vi "Configure RFSG.vi"(0 "Path in":refnum<class "SA 8GHz Path.lvclass">, 5 "Cal Point in":T1, 7 "External Gain":dbl, 9 "Digital Gain":dbl, 11 "error in (no error)":errorcluster) -> (4 "Path out":refnum<class "SA 8GHz Path.lvclass">, 6 "Cal Point out":T1, 15 "error out":errorcluster)   [LabVIEW 2023, in "RFFixtureCharact.RMM.lvlib" / "SA 8GHz Path.lvclass"]
uses:
  SA 8GHz Path.lvclass
  Public/Base Classes/Scalar/Scalar Path/Type Definitions/Cal Point.ctl
  <instrlib>/niRFSG/niRFSG.llb/niRFSG Ref Clock Sources.ctl
  SA 8GHz Path.lvclass/SA 8GHz Path.ctl
  Public/Base Classes/Scalar/Scalar Path/Scalar Path.lvclass
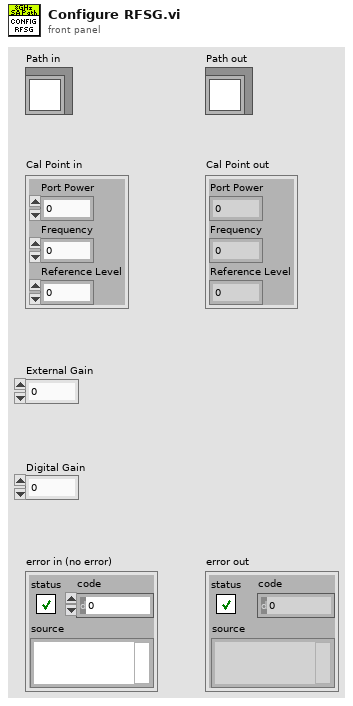
[diagram p1: front panel]
types:
  T1 = typedef "RFFixtureCharact.Public.lvlib/Scalar Path.lvclass/Cal Point.ctl" = cluster{"Port Power":dbl, "Frequency":dbl, "Reference Level":dbl}
  T2 = typedef "niRFSG Ref Clock Sources.ctl" = string
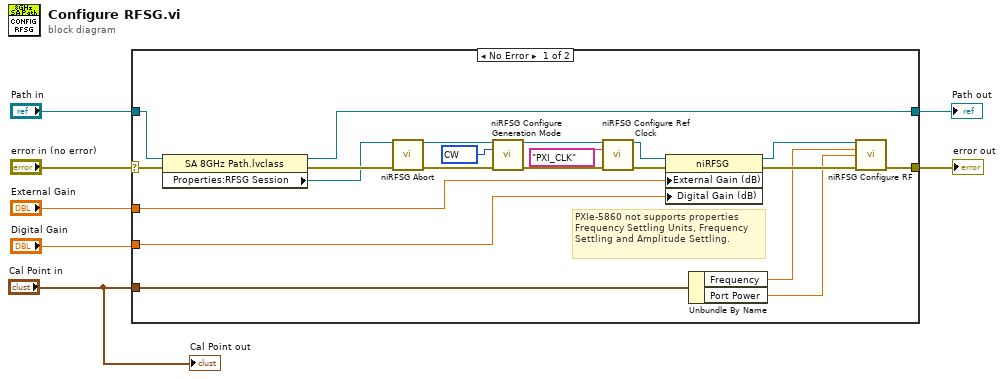
[diagram p0: block diagram]
diagram:
  n1 = case shown="No Error" "error in (no error)" {
    selector: "error in (no error)" -> [w17 w30]
    tunnel: [w18 w30] -> w4
    tunnel: [w10 w29] -> w6
    tunnel: "Path in" -> [w11 w29]
    tunnel: "Cal Point in" -> [w15 _]
    tunnel: "External Gain" -> [w12 _]
    tunnel: "Digital Gain" -> [w8 _]
    frame No Error {
      w22 = 1000 items=["CW"=1000, "Arb Waveform"=1001, "Script"=1002] ("generation mode")
      # "PXIe-5860 not supports properties Frequency Settling Units, Frequency Settling and Amplitude Settling."
      n2 = property class="SA 8GHz Path.lvclass"(reference=w11, error in=w17) -> (reference out=w10:refnum<class "SA 8GHz Path.lvclass">, error out=w19:errorcluster, "Properties:RFSG Session"=w9:refnum<k15>)
      n3 = call <instrlib>:"niRFSG Abort.vi"("instrument handle"=w9, "error in"=w19) -> ("instrument handle out"=w28:refnum<k15>, "error out"=w27:errorcluster)  [unwired: 12 in]
      n4 = call <instrlib>:"niRFSG Configure Generation Mode.vi"("instrument handle"=w28, "generation mode"=w22, "error in"=w27) -> ("instrument handle out"=w26:refnum<k15>, "error out"=w25:errorcluster)  [unwired: 11 in]
      n5 = call <instrlib>:"niRFSG Configure Ref Clock.vi"("instrument handle"=w26, "ref clock source"=T2 "PXI_CLK", "error in"=w25) -> ("instrument handle out"=w21:refnum<k15>, "error out"=w23:errorcluster)  [unwired: 11 in]
      n6 = property class="niRFSG"(reference=w21, error in=w23, "External Gain (dB)"=w12, "Digital Gain (dB)"=w8) -> (reference out=w20:refnum<k15>, error out=w16:errorcluster)
      n7 = Unbundle By Name(w15) -> ("Frequency"=w14:dbl, "Port Power"=w13:dbl)
      n8 = call <instrlib>:"niRFSG Configure RF.vi"("instrument handle"=w20, "frequency (Hz)"=w14, "power level (dBm)"=w13, "error in"=w16) -> ("error out"=w18:errorcluster)  [unwired: 10 in, 1 out]
    }
    frame Error {
    }
  }
  "error out" <- w4
  "Path out" <- w6
  "Cal Point out" <- "Cal Point in"
